vi "fgv_232_gnss.vi"(7 "cmd":enum16{"init", "read", "write", "close"}(ring), 8 "error in":errorcluster, 10 "write buff":string) -> (0 "error out":errorcluster, 1 "byte n":u32(graph), 3 "read_buffer":string)   [LabVIEW 2019]
uses:
  <vilib>/Instr/_visa.llb/VISA Configure Serial Port (Instr).vi
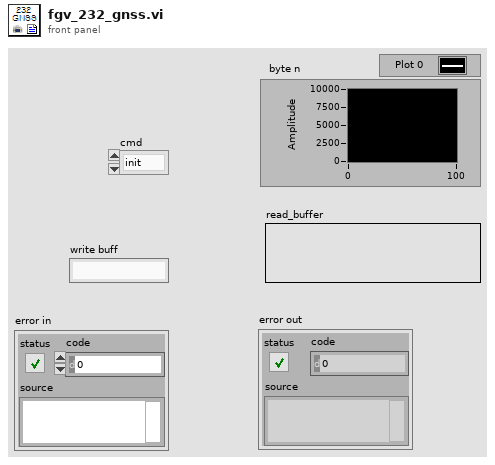
[diagram p1: front panel]
types:
  T1 = typedef "gnss_config.ctl" = cluster{"Port":refnum<visa-resource-name>, "heading select":string, "PwrPak7_mode select":string[], "rate":u32}
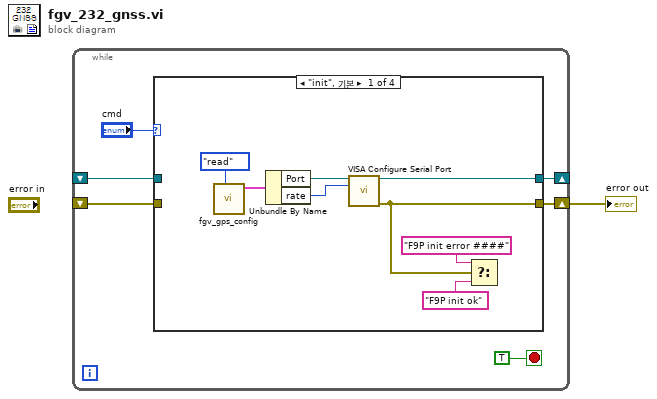
[diagram p0: block diagram]
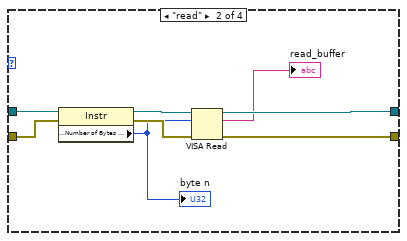
[diagram p2: hidden frame]
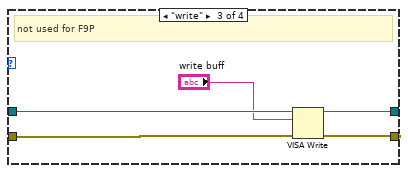
[diagram p3: hidden frame]
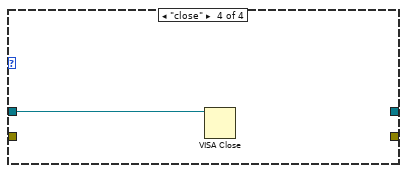
[diagram p4: hidden frame]
diagram:
  n1 = while {
    shift-right: [w5] -> _
    shift-left: _ -> [w3]
    shift-right: [w4] -> w1
    shift-left: _ -> [w2]
    stop <- TRUE stop-if-true
    n2 = case shown="\"init\", 기본" "cmd" {
      tunnel: [w15 w21 w26 _] -> w5
      tunnel: [w14 w20 w25 _] -> w4
      tunnel: w3 -> [_ w23 w27 w29]
      tunnel: w2 -> [_ w18 w28 _]
      frame "init", Default {
        n3 = call "fgv_gps_config.vi"("cmd"=enum16{"read", "write"}."read") -> ("GNSS cfg out"=w8:T1)  [unwired: 9 in, 1 out]
        n4 = Unbundle By Name(w8) -> ("Port"=w11:refnum<visa-resource-name>, "rate"=w10:u32)
        n5 = call-poly "VISA Configure Serial Port"("VISA resource name"=w11, "baud rate (9600)"=w10) -> ("VISA resource name out"=w15:refnum<visa-resource-name>, "error out"=w14:errorcluster)  [unwired: 12 in]
        n6 = Select(t="F9P init error ####" ("String in"), s=w14, f="F9P init ok" ("String in")) -> ()  [unwired: 1 out]
      }
      frame "read" {
        n7 = property class="Instr"(reference=w23, error in=w18) -> (reference out=w22:refnum<visa-resource-name>, error out=w19:errorcluster, "Serial Settings:Number of Bytes at Serial Port"=w16:u32)
        "byte n" <- w16
        n8 = VISA Read(VISA resource name=w22, byte count=w16, error in (no error)=w19) -> (VISA resource name out=w21:refnum<visa-resource-name>, read buffer=→"read_buffer":string, error out=w20:errorcluster)  [unwired: 1 out]
      }
      frame "write" {
        # "not used for F9P"
        n9 = VISA Write(VISA resource name=w27, write buffer="write buff", error in (no error)=w28) -> (VISA resource name out=w26:refnum<visa-resource-name>, error out=w25:errorcluster)  [unwired: 1 out]
      }
      frame "close" {
        n10 = VISA Close(VISA resource name=w29) -> ()  [unwired: 1 in, 1 out]
      }
    }
  }
  "error out" <- w1
